vi "BuildM2Sequence.vi"(8 "error in (no error)":errorcluster, 9 "Mode2 Test Properties":T2, 10 "Horizontal T deg":dbl=0.076 format="%#_13g", 11 "Sequence in":refnum<class "Sequence.lvclass">) -> (0 "error out":errorcluster, 2 "PAARD Test Seq":T4[](array[typedef])=[{"StepType"=enum."Motion", "RF In/Out"=enum."Rx - RF Out", "Module/Raster"=0, "Polarization"=enum."Horizontal", "AO-64 Array"=[], "Position"=[]}, {"StepType"=enum."RasterTest", "RF In/Out"=enum."Tx - RF In", "Module/Raster"=0, "Polarization"=enum."Vertical", "AO-64 Array"=[], "Position"=[]}, {"StepType"=enum."Motion", "RF In/Out"=enum."Rx - RF Out", "Module/Raster"=1, "Polarization"=enum."Horizontal", "AO-64 Array"=[], "Position"=[]}, {"StepType"=enum."RasterTest", "RF In/Out"=enum."Tx - RF In", "Module/Raster"=0, "Polarization"=enum."Vertical", "AO-64 Array"=[], "Position"=[]}, {"StepType"=enum."Motion", "RF In/Out"=enum."Rx - RF Out", "Module/Raster"=2, "Polarization"=enum."Horizontal", "AO-64 Array"=[], "Position"=[]}, {"StepType"=enum."RasterTest", "RF In/Out"=enum."Tx - RF In", "Module/Raster"=0, "Polarization"=enum."Vertical", "AO-64 Array"=[], "Position"=[]}, {"StepType"=enum."Motion", "RF In/Out"=enum."Rx - RF Out", "Module/Raster"=3, "Polarization"=enum."Horizontal", "AO-64 Array"=[], "Position"=[]}, {"StepType"=enum."RasterTest", "RF In/Out"=enum."Tx - RF In", "Module/Raster"=0, "Polarization"=enum."Vertical", "AO-64 Array"=[], "Position"=[]}, {"StepType"=enum."Motion", "RF In/Out"=enum."Rx - RF Out", "Module/Raster"=4, "Polarization"=enum."Horizontal", "AO-64 Array"=[], "Position"=[]}, {"StepType"=enum."RasterTest", "RF In/Out"=enum."Tx - RF In", "Module/Raster"=0, "Polarization"=enum."Vertical", "AO-64 Array"=[], "Position"=[]}, {"StepType"=enum."Motion", "RF In/Out"=enum."Rx - RF Out", "Module/Raster"=5, "Polarization"=enum."Horizontal", "AO-64 Array"=[], "Position"=[]}, {"StepType"=enum."RasterTest", "RF In/Out"=enum."Tx - RF In", "Module/Raster"=0, "Polarization"=enum."Vertical", "AO-64 Array"=[], "Position"=[]}, {"StepType"=enum."Motion", "RF In/Out"=enum."Rx - RF Out", "Module/Raster"=6, "Polarization"=enum."Horizontal", "AO-64 Array"=[], "Position"=[]}, {"StepType"=enum."RasterTest", "RF In/Out"=enum."Tx - RF In", "Module/Raster"=0, "Polarization"=enum."Vertical", "AO-64 Array"=[], "Position"=[]}, {"StepType"=enum."Motion", "RF In/Out"=enum."Rx - RF Out", "Module/Raster"=7, "Polarization"=enum."Horizontal", "AO-64 Array"=[], "Position"=[]}, {"StepType"=enum."RasterTest", "RF In/Out"=enum."Tx - RF In", "Module/Raster"=0, "Polarization"=enum."Vertical", "AO-64 Array"=[], "Position"=[]}, {"StepType"=enum."Motion", "RF In/Out"=enum."Rx - RF Out", "Module/Raster"=8, "Polarization"=enum."Horizontal", "AO-64 Array"=[], "Position"=[]}, {"StepType"=enum."RasterTest", "RF In/Out"=enum."Tx - RF In", "Module/Raster"=0, "Polarization"=enum."Vertical", "AO-64 Array"=[], "Position"=[]}, {"StepType"=enum."Motion", "RF In/Out"=enum."Rx - RF Out", "Module/Raster"=9, "Polarization"=enum."Horizontal", "AO-64 Array"=[], "Position"=[]}, {"StepType"=enum."RasterTest", "RF In/Out"=enum."Tx - RF In", "Module/Raster"=0, "Polarization"=enum."Vertical", "AO-64 Array"=[], "Position"=[]}, {"StepType"=enum."Motion", "RF In/Out"=enum."Rx - RF Out", "Module/Raster"=10, "Polarization"=enum."Horizontal", "AO-64 Array"=[], "Position"=[]}, {"StepType"=enum."RasterTest", "RF In/Out"=enum."Tx - RF In", "Module/Raster"=0, "Polarization"=enum."Vertical", "AO-64 Array"=[], "Position"=[]}, {"StepType"=enum."Motion", "RF In/Out"=enum."Rx - RF Out", "Module/Raster"=11, "Polarization"=enum."Horizontal", "AO-64 Array"=[], "Position"=[]}, {"StepType"=enum."RasterTest", "RF In/Out"=enum."Tx - RF In", "Module/Raster"=0, "Polarization"=enum."Vertical", "AO-64 Array"=[], "Position"=[]}, {"StepType"=enum."Motion", "RF In/Out"=enum."Rx - RF Out", "Module/Raster"=12, "Polarization"=enum."Horizontal", "AO-64 Array"=[], "Position"=[]}, {"StepType"=enum."RasterTest", "RF In/Out"=enum."Tx - RF In", "Module/Raster"=0, "Polarization"=enum."Vertical", "AO-64 Array"=[], "Position"=[]}, {"StepType"=enum."Motion", "RF In/Out"=enum."Rx - RF Out", "Module/Raster"=13, "Polarization"=enum."Horizontal", "AO-64 Array"=[], "Position"=[]}, {"StepType"=enum."RasterTest", "RF In/Out"=enum."Tx - RF In", "Module/Raster"=0, "Polarization"=enum."Vertical", "AO-64 Array"=[], "Position"=[]}, {"StepType"=enum."Motion", "RF In/Out"=enum."Rx - RF Out", "Module/Raster"=14, "Polarization"=enum."Horizontal", "AO-64 Array"=[], "Position"=[]}, {"StepType"=enum."RasterTest", "RF In/Out"=enum."Tx - RF In", "Module/Raster"=0, "Polarization"=enum."Vertical", "AO-64 Array"=[], "Position"=[]}, {"StepType"=enum."Motion", "RF In/Out"=enum."Rx - RF Out", "Module/Raster"=15, "Polarization"=enum."Horizontal", "AO-64 Array"=[], "Position"=[]}, {"StepType"=enum."RasterTest", "RF In/Out"=enum."Tx - RF In", "Module/Raster"=0, "Polarization"=enum."Vertical", "AO-64 Array"=[], "Position"=[]}, {"StepType"=enum."Motion", "RF In/Out"=enum."Rx - RF Out", "Module/Raster"=16, "Polarization"=enum."Horizontal", "AO-64 Array"=[], "Position"=[]}, {"StepType"=enum."RasterTest", "RF In/Out"=enum."Tx - RF In", "Module/Raster"=0, "Polarization"=enum."Vertical", "AO-64 Array"=[], "Position"=[]}, {"StepType"=enum."Motion", "RF In/Out"=enum."Rx - RF Out", "Module/Raster"=17, "Polarization"=enum."Horizontal", "AO-64 Array"=[], "Position"=[]}, {"StepType"=enum."RasterTest", "RF In/Out"=enum."Tx - RF In", "Module/Raster"=0, "Polarization"=enum."Vertical", "AO-64 Array"=[], "Position"=[]}, {"StepType"=enum."Motion", "RF In/Out"=enum."Rx - RF Out", "Module/Raster"=18, "Polarization"=enum."Horizontal", "AO-64 Array"=[], "Position"=[]}, {"StepType"=enum."RasterTest", "RF In/Out"=enum."Tx - RF In", "Module/Raster"=0, "Polarization"=enum."Vertical", "AO-64 Array"=[], "Position"=[]}, {"StepType"=enum."Motion", "RF In/Out"=enum."Rx - RF Out", "Module/Raster"=19, "Polarization"=enum."Horizontal", "AO-64 Array"=[], "Position"=[]}, {"StepType"=enum."RasterTest", "RF In/Out"=enum."Tx - RF In", "Module/Raster"=0, "Polarization"=enum."Vertical", "AO-64 Array"=[], "Position"=[]}, {"StepType"=enum."Finish", "RF In/Out"=enum."Tx - RF In", "Module/Raster"=0, "Polarization"=enum."Vertical", "AO-64 Array"=[], "Position"=[]}], 3 "Sequence out":refnum<class "Sequence.lvclass">, 5 "Axes to Move":T1[](array[typedef]))   [LabVIEW 2018, in "Sequence.lvclass"]
uses:
  Sequence.lvclass
  SequenceSubvis/mWaveTestStep.ctl
  SequenceSubvis/TestStepTypes.ctl
  SequenceSubvis/RF Direction.ctl
  SequenceSubvis/PolarizationSelect.ctl
  APARMainSubvis/VXM Public API/singleAxisMoveDef.ctl
  APARMainSubvis/VXM Public API/mmWaveAxis.ctl
  APARMainSubvis/UI temporary dialogs and VIs/Mode2TestProperties.ctl
  Sequence.lvclass/Sequence.ctl
  <vilib>/Utility/file.llb/Read Delimited Spreadsheet (DBL).vi
panel:
  out "Axes to Move 2":T1[](array[typedef])
  out "# steps":i32=41
  out "length, bytes":i32=1890 format="%.3p"
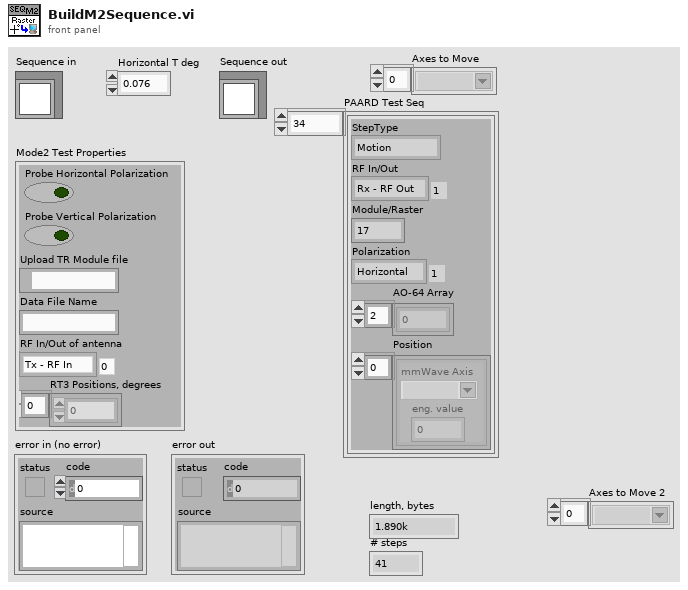
[diagram p1: front panel]
types:
  T1 = typedef "mmWaveAxis.ctl" = string
  T2 = typedef "Mode2TestProperties.ctl" = cluster{"Probe Horizontal Polarization":bool, "Probe Vertical Polarization":bool, "Upload TR Module file":path, "Data File Name":string, "RF In/Out of antenna":T3, "RT3 Positions, degrees":dbl[]}
  T3 = typedef "RF Direction.ctl" = enum16{"Tx - RF In", "Rx - RF Out"}
  T4 = typedef "mWaveTestStep.ctl" = cluster{"StepType":T5, "RF In/Out":T3, "Module/Raster":i32, "Polarization":T6, "AO-64 Array":dbl[], "Position":T7[]}
  T5 = typedef "TestStepTypes.ctl" = enum16{"MotionFF-M2", "Motion", "SweepTest", "RasterTest", "Finish", "64ModuleCfg"}
  T6 = typedef "PolarizationSelect.ctl" = enum16{"Vertical", "Horizontal"}
  T7 = typedef "singleAxisMoveDef.ctl" = cluster{"mmWave Axis":T1, "eng. value":dbl}
  T8 = typedef "Mode3FileRowData.ctl" = cluster{"X mm":dbl, "Y mm":dbl, "RT3, degrees":dbl, "sub-file path":path}
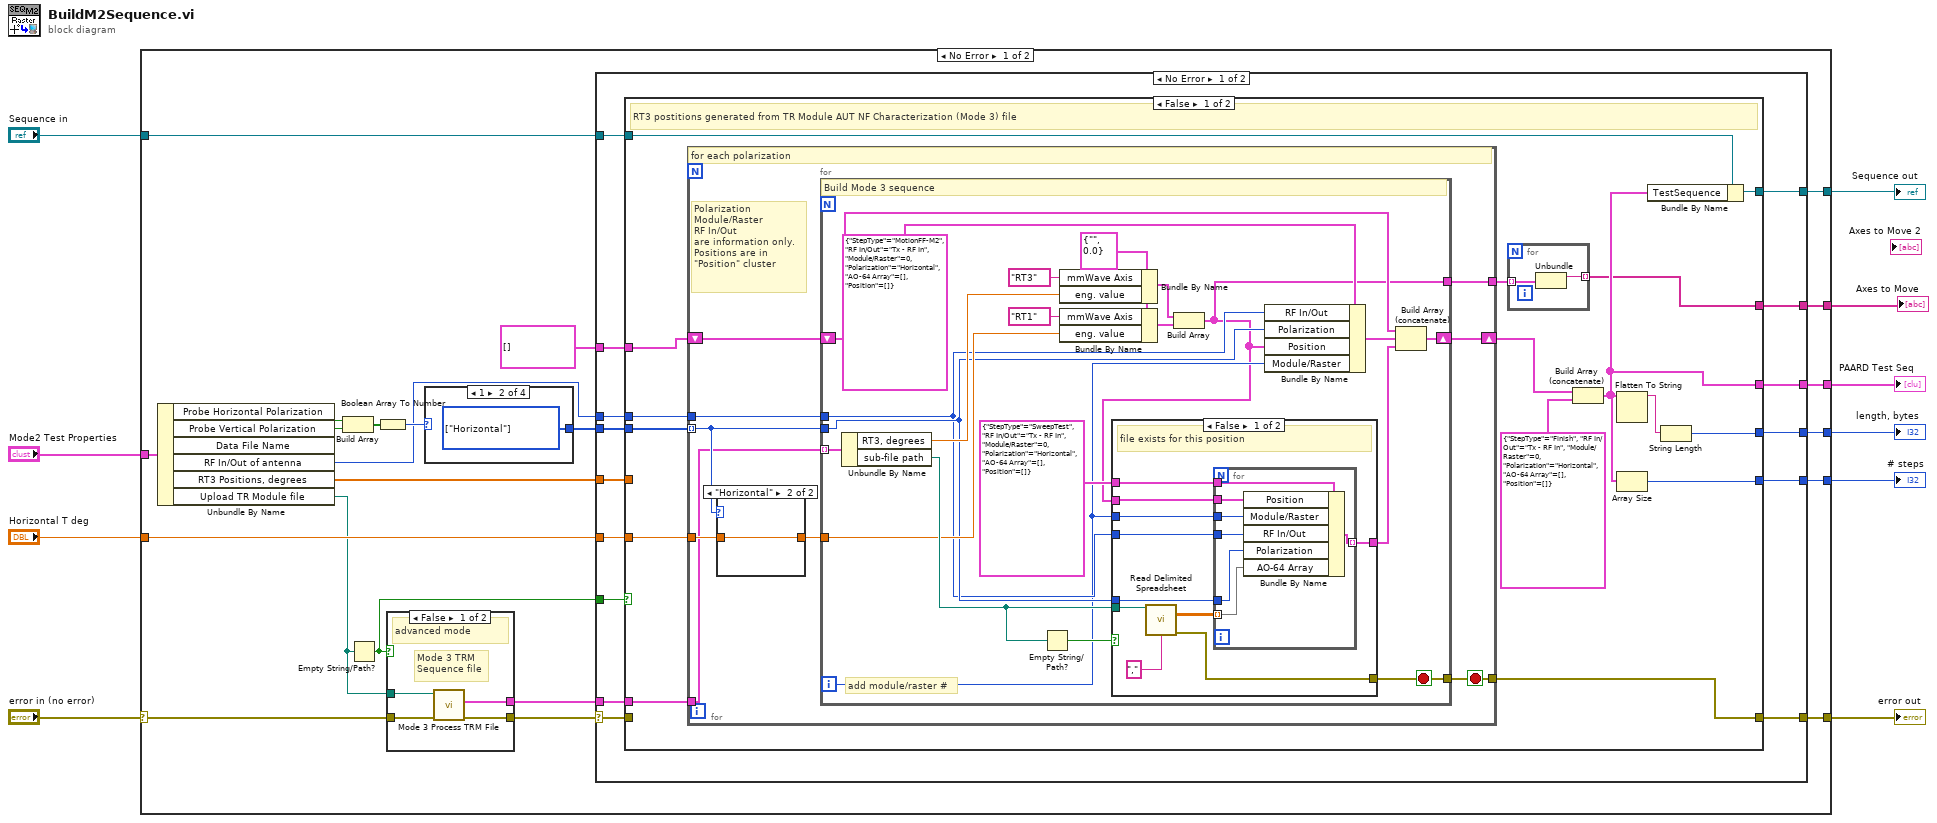
[diagram p0: block diagram]
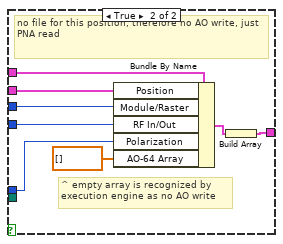
[diagram p2: hidden frame]
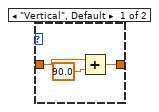
[diagram p3: hidden frame]
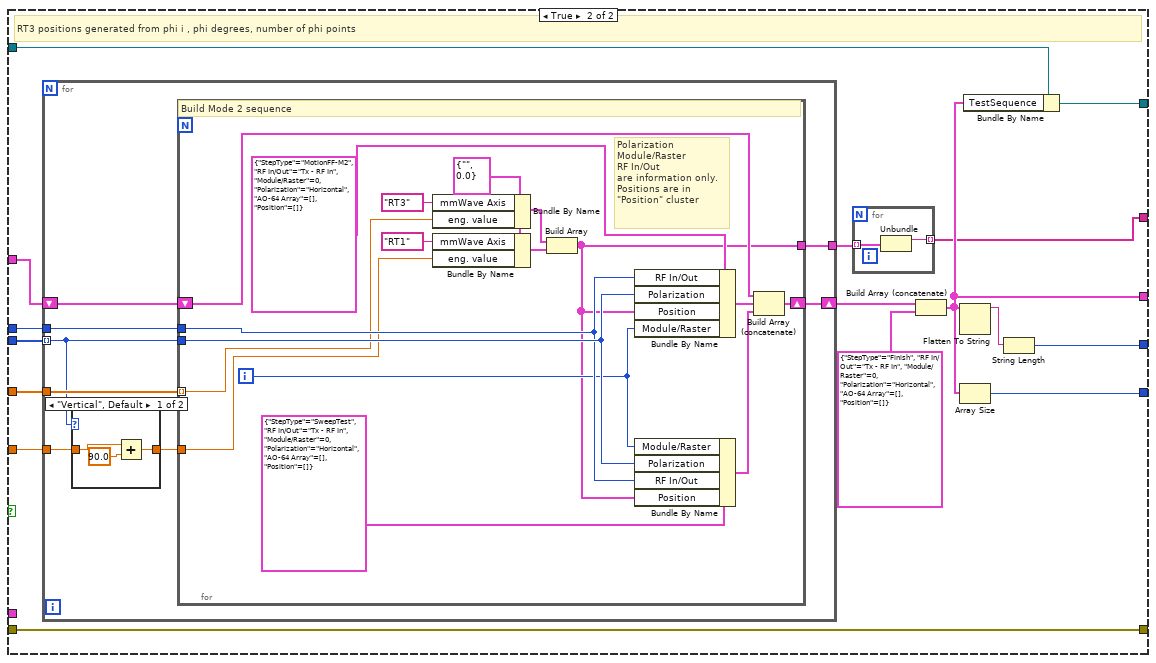
[diagram p4: hidden frame]
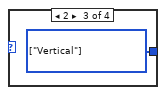
[diagram p9: hidden frame]
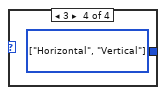
[diagram p10: hidden frame]
diagram:
  n1 = case shown="No Error" "error in (no error)" {
    selector: "error in (no error)" -> [w17 w183]
    tunnel: [w32 _] -> w10
    tunnel: [w18 _] -> w9
    tunnel: [w31 _] -> w8
    tunnel: "Mode2 Test Properties" -> [w29 _]
    tunnel: "Horizontal T deg" -> [w22 _]
    tunnel: [w14 w183] -> w5
    tunnel: "Sequence in" -> [w20 w182]
    tunnel: [w19 w182] -> w3
    tunnel: [w11 _] -> w1
    frame No Error {
      n2 = Unbundle By Name(w29) -> ("Probe Horizontal Polarization"=w28:bool, "Probe Vertical Polarization"=w27:bool, "RF In/Out of antenna"=w23:T3, "RT3 Positions, degrees"=w21:dbl[], "Upload TR Module file"=w16:path)  [unwired: 1 out]
      n3 = Build Array(w28, w27) -> (w26:bool[])
      n4 = Empty String/Path?(string/path=w16) -> (empty?=w12:bool)
      n5 = Boolean Array To Number(Boolean array=w26) -> (number=w25:u32)
      n6 = case shown="False" w12 {
        tunnel: w17 -> [w177 w178]
        tunnel: [w176 w178] -> w15
        tunnel: w16 -> [w175 _]
        tunnel: [w174 _] -> w13
        frame False {
          # "Mode 3 TRM\nSequence file"
          # "advanced mode"
          n7 = call "Mode 3 Process TRM File.vi"("error in (no error)"=w177, "Upload TR Module file"=w175) -> ("error out"=w176:errorcluster, "Mode 3 Steps"=w174:T8[])  [unwired: 7 in, 1 out]
        }
        frame True {
          # "\"standard\" mode"
        }
      }
      n8 = case shown="1" w25 {
        tunnel: [_ w179 w180 w181] -> w24
        frame 0, Default {
          # "should create an \nerror"
        }
        frame 1 {
          w179 = T6[] [enum."Horizontal"] items=["Vertical", "Horizontal"] ("Polarization(s)")
        }
        frame 2 {
          w180 = T6[] [enum."Vertical"] items=["Vertical", "Horizontal"] ("Polarization(s)")
        }
        frame 3 {
          w181 = T6[] [enum."Horizontal", enum."Vertical"] items=["Vertical", "Horizontal"] ("Polarization(s)")
        }
      }
      n9 = case shown="No Error" w15 {
        selector: w15 -> [w36 w173]
        tunnel: [w47 _] -> w32
        tunnel: [w46 _] -> w31
        tunnel: T4[] [] -> [w45 _]
        tunnel: w24 -> [w44 _]
        tunnel: w23 -> [w43 _]
        tunnel: w22 -> [w42 _]
        tunnel: w21 -> [w41 _]
        tunnel: w20 -> [w40 w172]
        tunnel: [w39 w172] -> w19
        tunnel: [w38 _] -> w18
        tunnel: [w35 w173] -> w14
        tunnel: w13 -> [w37 _]
        tunnel: w12 -> [w34 _]
        tunnel: [w33 _] -> w11
        frame No Error {
          n10 = case shown="False" w34 {
            tunnel: [w55 w139] -> w47
            tunnel: [w54 w138] -> w46
            tunnel: w45 -> [w57 w137]
            tunnel: w44 -> [w59 w135]
            tunnel: w43 -> [w58 w134]
            tunnel: w42 -> [w56 w133]
            tunnel: w41 -> [_ w132]
            tunnel: w40 -> [w51 w130]
            tunnel: [w52 w129] -> w39
            tunnel: [w50 w127] -> w38
            tunnel: w37 -> [w60 _]
            tunnel: [w53 w128] -> w35
            tunnel: w36 -> [_ w128]
            tunnel: [w48 w125] -> w33
            frame False {
              # "RT3 postitions generated from TR Module AUT NF Characterization (Mode 3) file"
              n11 = for {
                tunnel: w58 -> [w70]
                tunnel: w56 -> [w74]
                shift-right: [w72] -> w63
                shift-left: w57 -> [w71]
                tunnel: w59 -> [w69] mode=indexing
                tunnel: [w68] -> w53
                tunnel: w60 -> [w67]
                tunnel: [w66] -> w49
                stop <- w68 stop-if-true
                # "Polarization\nModule/Raster\nRF In/Out\nare information only.\nPositions are in \n\"Position\" cluster"
                # "for each polarization"
                n12 = case shown="\"Horizontal\"" w69 {
                  tunnel: [w123 w124] -> w73
                  tunnel: w74 -> [w122 w124]
                  frame "Vertical", Default {
                    n13 = Add(x=w122, y=90.0) -> (x+y=w123:dbl)
                  }
                  frame "Horizontal" {
                  }
                }
                n14 = for {
                  tunnel: w67 -> [w95] mode=indexing
                  shift-right: [w94] -> w72
                  shift-left: w71 -> [w87]
                  tunnel: w73 -> [w79]
                  tunnel: w70 -> [w77]
                  tunnel: w69 -> [w78]
                  tunnel: [w86] -> w68
                  tunnel: [w75] -> w66
                  i -> [w76]
                  stop <- w86 stop-if-true
                  w85 = T7 {"mmWave Axis"="", "eng. value"=0.0} ("Move")
                  # "add module/raster #"
                  # "Build Mode 3 sequence"
                  n15 = Unbundle By Name(w95) -> ("RT3, degrees"=w80:dbl, "sub-file path"=w88:path)
                  n16 = Empty String/Path?(string/path=w88) -> (empty?=w92:bool)
                  n17 = Bundle By Name(cluster=w85, "mmWave Axis"=T1 "RT3", "eng. value"=w80) -> (w82:T7)
                  n18 = Bundle By Name(cluster=w85, "mmWave Axis"=T1 "RT1", "eng. value"=w79) -> (w81:T7)
                  n19 = Build Array(w82, w81) -> (w75:T7[])
                  n20 = case shown="False" w92 {
                    tunnel: T4 {"StepType"=enum."SweepTest", "RF In/Out"=enum."Tx - RF In", "Module/Raster"=0, "Polarization"=enum."Horizontal", "AO-64 Array"=[], "Position"=[]} ("Test") -> [w105 w120]
                    tunnel: w77 -> [w104 w119]
                    tunnel: w78 -> [w102 w118]
                    tunnel: [w101 w115] -> w93
                    tunnel: w88 -> [w100 _]
                    tunnel: w76 -> [w98 w114]
                    tunnel: [w97 _] -> w86
                    tunnel: w75 -> [w96 w113]
                    frame False {
                      # "file exists for this position"
                      n21 = call-poly <vilib>:"Read Delimited Spreadsheet.vi"("file path (dialog if empty)"=w100, "delimiter (\\t)"="," ("delimiter (\\t)")) -> ("all rows"=w103:dbl[][], "error out"=w97:errorcluster)  [unwired: 8 in, 4 out]
                      n22 = for {
                        tunnel: w105 -> [w112]
                        tunnel: w104 -> [w111]
                        tunnel: w103 -> [w110] mode=indexing
                        tunnel: w102 -> [w109]
                        tunnel: [w108] -> w101 mode=indexing
                        tunnel: w98 -> [w107]
                        tunnel: w96 -> [w106]
                        n23 = Bundle By Name(cluster=w112, "Position"=w106, "Module/Raster"=w107, "RF In/Out"=w111, "Polarization"=w109, "AO-64 Array"=w110) -> (w108:T4)
                      }
                    }
                    frame True {
                      # "^ empty array is recognized by \nexecution engine as no AO write"
                      # "no file for this position, therefore no AO write, just PNA read"
                      n24 = Bundle By Name(cluster=w120, "Position"=w113, "Module/Raster"=w114, "RF In/Out"=w119, "Polarization"=w118, "AO-64 Array"=dbl[] []) -> (w116:T4)
                      n25 = Build Array(w116) -> (w115:T4[])
                    }
                  }
                  n26 = Bundle By Name(cluster=T4 {"StepType"=enum."MotionFF-M2", "RF In/Out"=enum."Tx - RF In", "Module/Raster"=0, "Polarization"=enum."Horizontal", "AO-64 Array"=[], "Position"=[]} ("Test"), "RF In/Out"=w77, "Polarization"=w78, "Position"=w75, "Module/Raster"=w76) -> (w91:T4)
                  n27 = Build Array (concatenate)(w87, w91, w93) -> (w94:T4[])
                }
              }
              n28 = for {
                tunnel: w49 -> [w65] mode=indexing
                tunnel: [w64] -> w48 mode=indexing
                n29 = Unbundle(w65) -> ("mmWave Axis"=w64:T1)  [unwired: 1 out]
              }
              n30 = Build Array (concatenate)(w63, T4 {"StepType"=enum."Finish", "RF In/Out"=enum."Tx - RF In", "Module/Raster"=0, "Polarization"=enum."Horizontal", "AO-64 Array"=[], "Position"=[]} ("Test")) -> (w50:T4[])
              n31 = Flatten To String(anything=w50) -> (data string=w61:string)  [unwired: 3 in, 2 out]
              n32 = Array Size(array=w50) -> (size(s)=w54:i32)
              n33 = Bundle By Name(cluster=w51, "TestSequence"=w50) -> (w52:refnum<class "Sequence.lvclass">)
              n34 = String Length(string=w61) -> (length=w55:i32)
            }
            frame True {
              # "RT3 positions generated from phi i , phi degrees, number of phi points"
              n35 = for {
                tunnel: w134 -> [w150]
                tunnel: w132 -> [w149]
                tunnel: w133 -> [w145]
                shift-right: [w148] -> w136
                shift-left: w137 -> [w147]
                tunnel: w135 -> [w146] mode=indexing
                tunnel: [w143] -> w126
                n36 = case shown="\"Vertical\", Default" w146 {
                  tunnel: [w153 w154] -> w144
                  tunnel: w145 -> [w152 w154]
                  frame "Vertical", Default {
                    n37 = Add(x=w152, y=90.0) -> (x+y=w153:dbl)
                  }
                  frame "Horizontal" {
                  }
                }
                n38 = for {
                  tunnel: w150 -> [w165]
                  tunnel: w146 -> [w166]
                  tunnel: w149 -> [w158] mode=indexing
                  shift-right: [w170] -> w148
                  shift-left: w147 -> [w169]
                  tunnel: w144 -> [w157]
                  tunnel: [w155] -> w143
                  i -> [w156]
                  w163 = T7 {"mmWave Axis"="", "eng. value"=0.0} ("Move")
                  # "Polarization\nModule/Raster\nRF In/Out\nare information only.\nPositions are in \n\"Position\" cluster"
                  # "Build Mode 2 sequence"
                  n39 = Bundle By Name(cluster=w163, "mmWave Axis"=T1 "RT3", "eng. value"=w158) -> (w160:T7)
                  n40 = Bundle By Name(cluster=w163, "mmWave Axis"=T1 "RT1", "eng. value"=w157) -> (w159:T7)
                  n41 = Build Array(w160, w159) -> (w155:T7[])
                  n42 = Bundle By Name(cluster=T4 {"StepType"=enum."MotionFF-M2", "RF In/Out"=enum."Tx - RF In", "Module/Raster"=0, "Polarization"=enum."Horizontal", "AO-64 Array"=[], "Position"=[]} ("Test"), "RF In/Out"=w165, "Polarization"=w166, "Position"=w155, "Module/Raster"=w156) -> (w171:T4)
                  n43 = Bundle By Name(cluster=T4 {"StepType"=enum."SweepTest", "RF In/Out"=enum."Tx - RF In", "Module/Raster"=0, "Polarization"=enum."Horizontal", "AO-64 Array"=[], "Position"=[]} ("Test"), "Module/Raster"=w156, "Polarization"=w166, "RF In/Out"=w165, "Position"=w155) -> (w167:T4)
                  n44 = Build Array (concatenate)(w169, w171, w167) -> (w170:T4[])
                }
              }
              n45 = for {
                tunnel: w126 -> [w142] mode=indexing
                tunnel: [w141] -> w125 mode=indexing
                n46 = Unbundle(w142) -> ("mmWave Axis"=w141:T1)  [unwired: 1 out]
              }
              n47 = Build Array (concatenate)(w136, T4 {"StepType"=enum."Finish", "RF In/Out"=enum."Tx - RF In", "Module/Raster"=0, "Polarization"=enum."Horizontal", "AO-64 Array"=[], "Position"=[]} ("Test")) -> (w127:T4[])
              n48 = Flatten To String(anything=w127) -> (data string=w140:string)  [unwired: 3 in, 2 out]
              n49 = Array Size(array=w127) -> (size(s)=w138:i32)
              n50 = Bundle By Name(cluster=w130, "TestSequence"=w127) -> (w129:refnum<class "Sequence.lvclass">)
              n51 = String Length(string=w140) -> (length=w139:i32)
            }
          }
        }
        frame Error {
        }
      }
    }
    frame Error {
    }
  }
  "error out" <- w5
  "Sequence out" <- w3
  "PAARD Test Seq" <- w9
  "length, bytes" <- w10
  "# steps" <- w8
  "Axes to Move" <- w1
